vi "Rational Interpolation.vi"(3 "x value":dbl format="%0.2f", 4 "X":dbl[](array[numeric]) format="%0.2f", 5 "Y":dbl[](array[numeric]) format="%0.2f") -> (0 "error":i32, 1 "interpolation error":dbl format="%0.2f", 2 "interpolation value":dbl format="%0.2f")   [LabVIEW 2020, in "NI_AALPro.lvlib"]
doc: "Interpolates or extrapolates f at <B>x value</B> using a rational function. The rational function passes through all the points formed by <B>Y</B> and <B>X</B>."
uses:
  NI_AALPro.lvlib
  <resource>/lvanlys.dll
panel:
  # "Rational Interpolation"
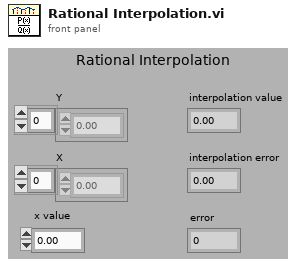
[diagram p1: front panel]
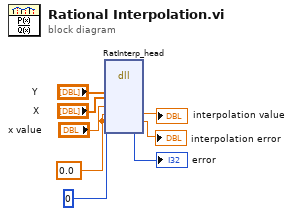
[diagram p0: block diagram]
diagram:
  w2 = 0.0
  n1 = dll-call lib="C:/Program Files (x86)/National Instruments/LabVIEW 2020/resource/lvanlys.*" fn="RatInterp_head"("Y"="Y", "X"="X", "x value"="x value", "output param"=w2, "output param"=w2, "output param"=0) -> ("output param"=→"interpolation value":dbl, "output param"=→"interpolation error":dbl, "output param"=→"error":i32)  [unwired: 7 in, 2 out]
